vi "Analog PassFail (SubVI).vi"(0 "MulticolumnListbox in":refnum<vi>, 1 "Array IN":refnum<vi>, 5 "row":i32, 7 "Array(F)/MC(T)":bool=TRUE, 9 "ResultInput":string, 11 "error in (no error)":errorcluster, 12 "String in":refnum<vi>, 13 "ATP(T)/FTP(F)":bool) -> (6 "Test Pass(F)Fail(T)?":bool, 15 "error out":errorcluster)   [LabVIEW 2017]
uses:
  <vilib>/Utility/miscctls.llb/LVRowAndColumnTypeDef.ctl
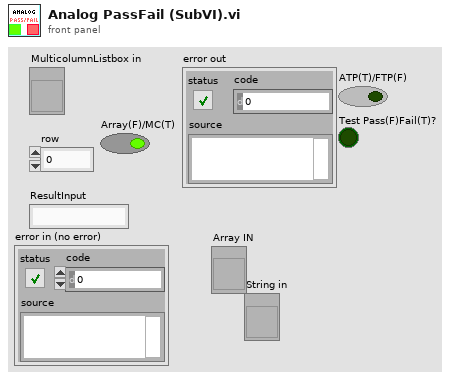
[diagram p1: front panel]
types:
  T1 = typedef "LVRowAndColumnTypeDef.ctl" = cluster{"Row":i32, "Column":i32}
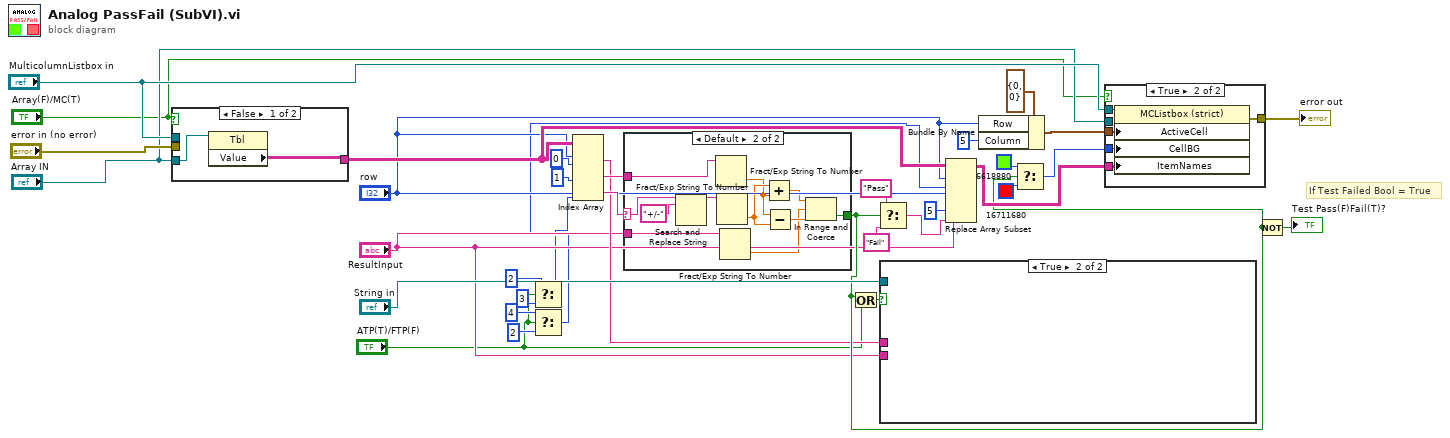
[diagram p0: block diagram]
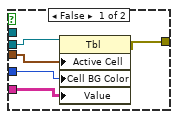
[diagram p2: hidden frame]
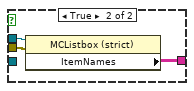
[diagram p3: hidden frame]
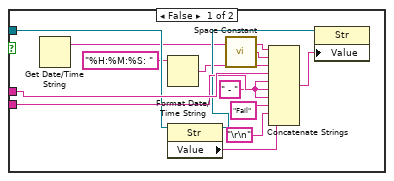
[diagram p4: hidden frame]
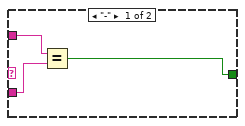
[diagram p5: hidden frame]
diagram:
  # "If Test Failed Bool = True"
  n1 = case shown="False" "Array(F)/MC(T)" {
    tunnel: [w36 w40] -> w25
    tunnel: "MulticolumnListbox in" -> [_ w39]
    tunnel: "error in (no error)" -> [_ w38]
    tunnel: "Array IN" -> [w37 _]
    frame False {
      n2 = property class="Tbl"(reference=w37) -> ("Value"=w36:string[][])  [unwired: 1 in, 2 out]
    }
    frame True {
      n3 = property class="MCListbox (strict)"(reference=w39, error in=w38) -> ("ItemNames"=w40:string[][])  [unwired: 2 out]
    }
  }
  n4 = Select(t=2, s="ATP(T)/FTP(F)", f=3 ("disabled index (col)")) -> (s? t:f=w4:i32)
  n5 = Select(t=4, s="ATP(T)/FTP(F)", f=2 ("disabled index (col)")) -> (s? t:f=w7:i32)
  n6 = Index Array(array=w25, index (row) #1="row", index (col) #1=0 ("disabled index (col)"), index (row) #2="row", index (col) #2=1 ("index (row)"), index (row) #3="row", index (col) #3=w4) -> (element #1=w14:string, element #2=w22:string, element #3=w19:string)
  n7 = case shown="Default" w19 {
    selector: w19 -> [_ w52]
    tunnel: "ResultInput" -> [w42 w48]
    tunnel: w22 -> [w43 w46]
    tunnel: [w41 w44] -> w15
    frame "-" {
      n8 = Equal?(x=w43, y=w42) -> (x = y?=w41:bool)
    }
    frame Default {
      n9 = Search and Replace String(input string=w52, search string="+/-") -> (result string=w53:string)  [unwired: 6 in, 3 out]
      n10 = Fract/Exp String To Number(string=w46) -> (number=w45:dbl)  [unwired: 3 in, 1 out]
      n11 = Fract/Exp String To Number(string=w53) -> (number=w49:dbl)  [unwired: 3 in, 1 out]
      n12 = Fract/Exp String To Number(string=w48) -> (number=w47:dbl)  [unwired: 3 in, 1 out]
      n13 = Add(x=w49, y=w45) -> (x+y=w50:dbl)
      n14 = Subtract(x=w45, y=w49) -> (x-y=w51:dbl)
      n15 = In Range and Coerce(upper limit=w50, x=w47, lower limit=w51) -> (In Range?=w44:bool)  [unwired: 1 out]
    }
  }
  n16 = Or(x=w15, y="ATP(T)/FTP(F)") -> (x .or. y?=w9:bool)
  n17 = Select(t="Pass", s=w15, f="Fail") -> (s? t:f=w27:string)
  n18 = case shown="True" w9 {
    tunnel: "String in" -> [w61 _]
    tunnel: w14 -> [w67 _]
    tunnel: "ResultInput" -> [w66 _]
    frame False {
      w65 = " - " ("string")
      n19 = Get Date/Time String() -> (date string=w56:string)  [unwired: 3 in, 1 out]
      n20 = Format Date/Time String(time format string (%c)="%H:%M:%S: ") -> (date/time string=w57:string)  [unwired: 2 in]
      n21 = property class="Str"(reference=w61) -> (reference out=w60:refnum<vi>, "Value"=w59:string)  [unwired: 1 in, 1 out]
      n22 = call <vilib>:"Space Constant.vi"() -> ("String"=w55:string)
      n23 = Concatenate Strings(w56, w55, w57, w67, w65, w66, w65, "Fail" ("string"), "\r\n", w59) -> (w62:string)
      n24 = property class="Str"(reference=w60, "Value"=w62) -> ()  [unwired: 1 in, 2 out]
    }
    frame True {
    }
  }
  n25 = Replace Array Subset(array=w25, new element #1="ResultInput", index (row) #1="row", index (col) #1=w7, new element #2=w27, index (row) #2="row", index (col) #2=5 ("disabled index (col)")) -> (w34:string[][])
  n26 = Bundle By Name(cluster=T1 {"Row"=0, "Column"=0} ("Active Cell:Active Cell"), "Row"="row", "Column"=5) -> (w29:T1)
  n27 = Select(t=u32 6618880, s=w15, f=u32 16711680) -> (s? t:f=w33:u32)
  n28 = case shown="True" "Array(F)/MC(T)" {
    tunnel: [w71 w77] -> w35
    tunnel: w34 -> [w68 w76]
    tunnel: w33 -> [w69 w75]
    tunnel: w29 -> [w70 w74]
    tunnel: "MulticolumnListbox in" -> [_ w73]
    tunnel: "Array IN" -> [w72 _]
    frame False {
      n29 = property class="Tbl"(reference=w72, "Active Cell"=w70, "Cell BG Color"=w69, "Value"=w68) -> (error out=w71:errorcluster)  [unwired: 1 in, 1 out]
    }
    frame True {
      n30 = property class="MCListbox (strict)"(reference=w73, "ActiveCell"=w74, "CellBG"=w75, "ItemNames"=w76) -> (error out=w77:errorcluster)  [unwired: 1 in, 1 out]
    }
  }
  "error out" <- w35
  n31 = Not(x=w15) -> (.not. x?=→"Test Pass(F)Fail(T)?":bool)
